vi "controller.vi"(8 "error in (no error)":errorcluster, 11 "Message Queues":T1) -> (0 "error out":errorcluster)   [LabVIEW 2015]
uses:
  support/Message Queue/Message Queue.lvlib
  support/Message Queue/Message Cluster.ctl
  support/Message Queue/All Message Queues.ctl
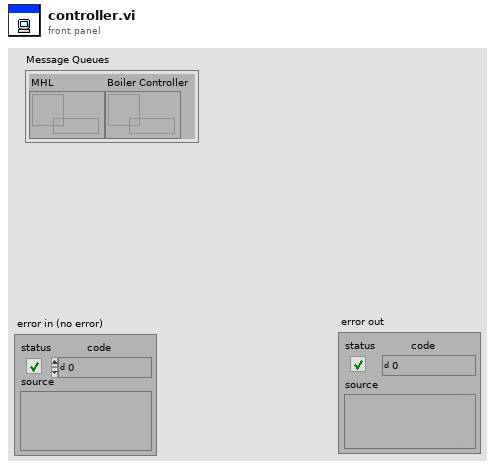
[diagram p1: front panel]
types:
  T1 = typedef "Message Queue.lvlib/All Message Queues.ctl" = cluster{"MHL":refnum<queue>, "Boiler Controller":refnum<queue>}
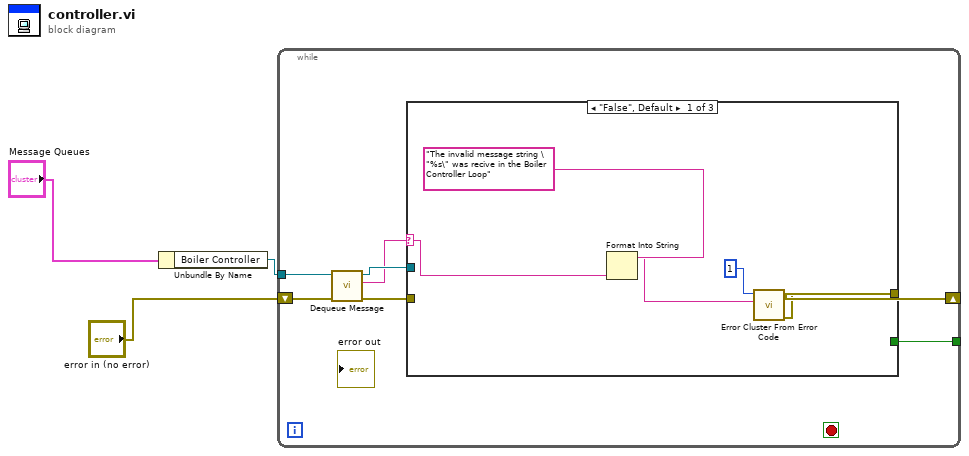
[diagram p0: block diagram]
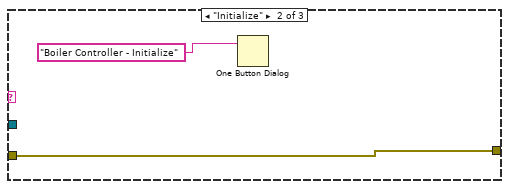
[diagram p2: hidden frame]
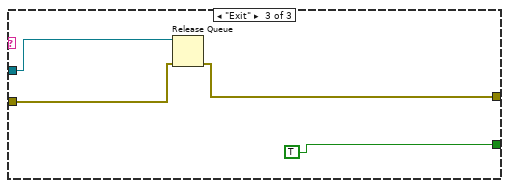
[diagram p3: hidden frame]
diagram:
  n1 = Unbundle By Name("Message Queues") -> ("Boiler Controller"=w2:refnum<queue>)
  n2 = while {
    tunnel: w2 -> [w10]
    shift-right: [w5] -> _
    shift-left: "error in (no error)" -> [w9]
    tunnel: [w4] -> _
    stop <- _ stop-if-true
    n3 = call "Dequeue Message.vi"("error in (no error)"=w9, "Message Queue"=w10) -> ("error out"=w6:errorcluster, "Message"=w7:string, "dup Message Queue"=w8:refnum<queue>)  [unwired: 6 in, 1 out]
    n4 = case shown="\"False\", Default" w7 {
      selector: w7 -> [w14 _ _]
      tunnel: w8 -> [_ _ w21]
      tunnel: [w11 w17 w19] -> w5
      tunnel: w6 -> [_ w17 w20]
      tunnel: [_ _ TRUE] -> w4
      frame "False", Default {
        n5 = Format Into String(initial string="The invalid message string \"%s\" was recive in the Boiler Controller Loop", w14) -> (resulting string=w13:string)  [unwired: 2 in, 1 out]
        n6 = call <vilib>:"Error Cluster From Error Code.vi"("error message (\"\")"=w13, "error code (0)"=1) -> ("error out"=w11:errorcluster)  [unwired: 7 in]
      }
      frame "Initialize" {
        n7 = One Button Dialog(message="Boiler Controller - Initialize") -> ()  [unwired: 1 in, 1 out]
      }
      frame "Exit" {
        n8 = Release Queue(queue=w21, error in (no error)=w20) -> (error out=w19:errorcluster)  [unwired: 1 in, 2 out]
      }
    }
  }
